vi "write_params.vi"(8 "error in (no error)":errorcluster, 10 "params":T1={"criterion"="mse", "splitter"="random", "max_depth"={"max_depth_type"="None", "max_depth_int"=0.0}, "min_samples_split"=2.0, "min_samples_leaf"=1.0, "min_weight_fraction_leaf"=0.0, "max_features"={"max_features_type"="None", "max_features_int"=0.0, "max_features_float"=0.0}, "random_state"=0.0, "max_leaf_nodes"={"max_leaf_nodes_type"="None", "max_leaf_nodes_int"=100.0}, "min_impurity_decrease"=0.0, "ccp_alpha"=0.0}, 11 "DecisionTreeRegressor in":refnum<class "DecisionTreeRegressor.lvclass">) -> (0 "error out":errorcluster, 3 "DecisionTreeRegressor out":refnum<class "DecisionTreeRegressor.lvclass">)   [LabVIEW 2020, in "DecisionTreeRegressor.lvclass"]
uses:
  DecisionTreeRegressor.lvclass
  Controls/decision_tree_regressor_params.ctl
  DecisionTreeRegressor.lvclass/DecisionTreeRegressor.ctl
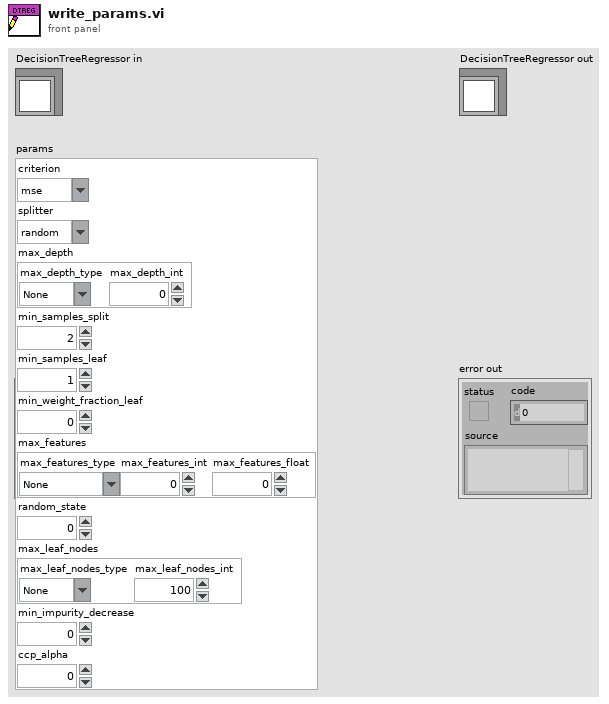
[diagram p1: front panel]
types:
  T1 = typedef "decision_tree_regressor_params.ctl" = cluster{"criterion":string, "splitter":string, "max_depth":cluster{"max_depth_type":string, "max_depth_int":dbl}, "min_samples_split":dbl, "min_samples_leaf":dbl, "min_weight_fraction_leaf":dbl, "max_features":cluster{"max_features_type":string, "max_features_int":dbl, "max_features_float":dbl}, "random_state":dbl, "max_leaf_nodes":cluster{"max_leaf_nodes_type":string, "max_leaf_nodes_int":dbl}, "min_impurity_decrease":dbl, "ccp_alpha":dbl}
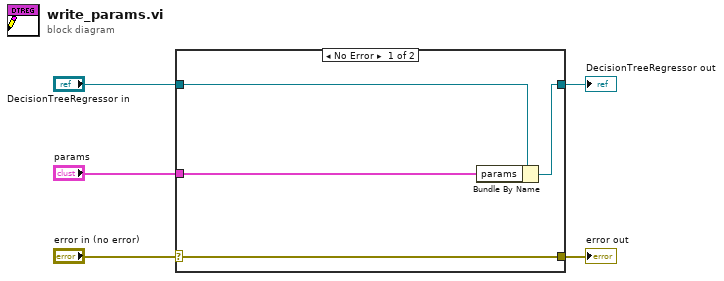
[diagram p0: block diagram]
diagram:
  n1 = case shown="No Error" "error in (no error)" {
    selector: "error in (no error)" -> [w9 w10]
    tunnel: [w9 w10] -> w4
    tunnel: [w7 w11] -> w2
    tunnel: "DecisionTreeRegressor in" -> [w8 w11]
    tunnel: "params" -> [w6 _]
    frame No Error {
      n2 = Bundle By Name(cluster=w8, "params"=w6) -> (w7:refnum<class "DecisionTreeRegressor.lvclass">)
    }
    frame Error {
    }
  }
  "error out" <- w4
  "DecisionTreeRegressor out" <- w2
